vi "ULx Create 1D Digital  Waveform.vi"(0 "t0":ext format="%#_10g", 5 "dt":dbl, 7 "data List":refnum<k24>, 11 "error in":errorcluster) -> (4 "data":digitalwaveform[](array[waveform]), 15 "error out":errorcluster)   [LabVIEW 2020]
uses:
  C:/Users/William/Documents/LV 2020 builds/LeaktestDAQ/Source-v33/ULx_LV.dll
  ULx_LV.dll
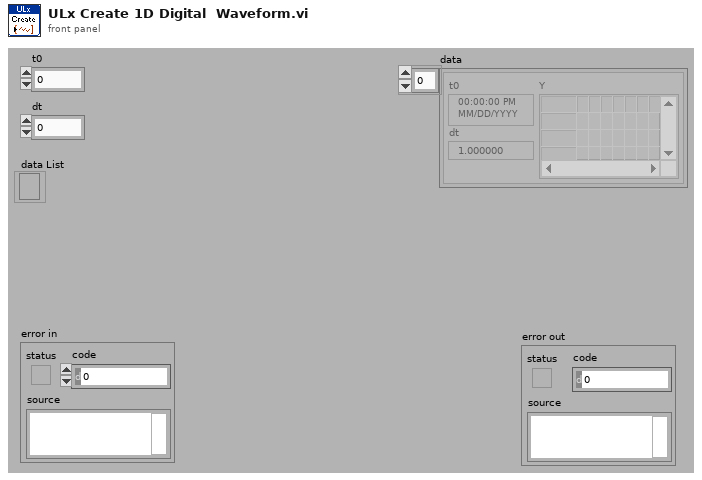
[diagram p1: front panel]
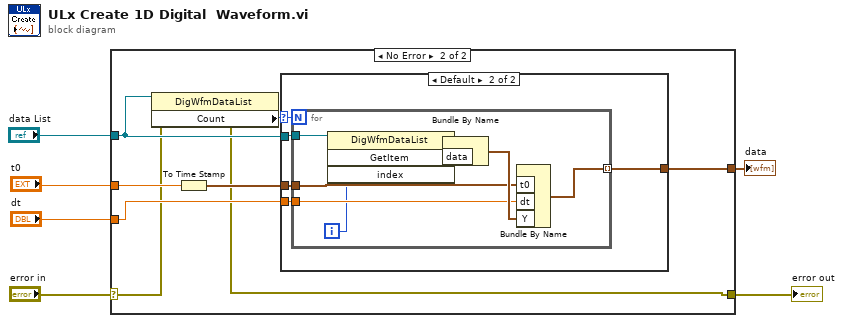
[diagram p0: block diagram]
diagram:
  n1 = case shown="No Error" "error in" {
    selector: "error in" -> [w7 w9]
    tunnel: [w7 w8] -> w5
    tunnel: "t0" -> [_ w15]
    tunnel: "dt" -> [_ w10]
    tunnel: "data List" -> [_ w13]
    tunnel: [_ w12] -> w1
    frame Error {
    }
    frame No Error {
      n2 = property class="DigWfmDataList"(reference=w13, error in=w9) -> (error out=w8:errorcluster, "Count"=w14:i32)  [unwired: 1 out]
      n3 = To Time Stamp(1:w15) -> (0:w11:timestamp)
      n4 = case shown="Default" w14 {
        selector: w14 -> [_ w20]
        tunnel: w13 -> [_ w19]
        tunnel: [_ w18] -> w12
        tunnel: w11 -> [_ w17]
        tunnel: w10 -> [_ w16]
        frame 0 {
        }
        frame Default {
          n5 = for {
            N: w20 -> [_]
            tunnel: w19 -> [w27]
            tunnel: [w24] -> w18 mode=indexing
            tunnel: w17 -> [w23]
            tunnel: w16 -> [w22]
            i -> [w21]
            n6 = invoke class="DigWfmDataList" method="GetItem"(reference=w27, "index"=w21) -> ("GetItem"=w26:u8[][])  [unwired: 2 in, 3 out]
            n7 = Bundle By Name("data"=w26) -> (w25:digitaldata)  [unwired: 1 in]
            n8 = Bundle By Name("t0"=w23, "dt"=w22, "Y"=w25) -> (w24:digitalwaveform)  [unwired: 1 in]
          }
        }
      }
    }
  }
  "error out" <- w5
  "data" <- w1
